vi "전체적인 좌표변환 구조.vi"() -> ()   [LabVIEW 2016]
panel:
  out "Lane":dbl[][](array[numeric])
  out "Obstacle":dbl[][](array[numeric])
  in  "IMU Data":string
  in  "Platform Data":string
  in  "NMEA Data":string
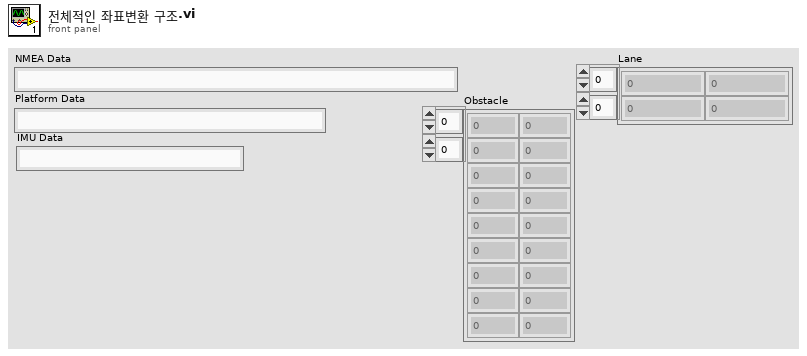
[diagram p1: front panel]
types:
  T1 = cluster{"GPS_Time":string, "GPS_Date":string, "GPS_N/S":string, "GPS_E/W":string, "GPS Raw_Lat":dbl, "GPS Raw_Lon":dbl, "GPS Raw_Speed [m/s]":dbl, "GPS Raw_Speed [km/h]":dbl, "GPS Raw_Bearing angle":dbl, "Checksum":bool, "Validity":bool}
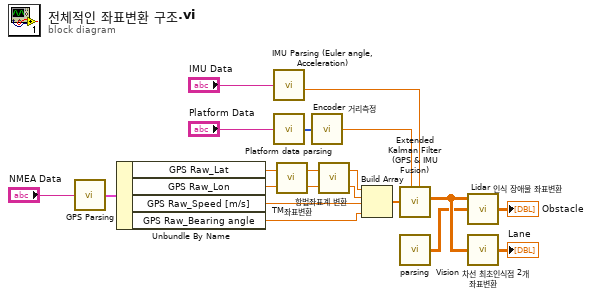
[diagram p0: block diagram]
diagram:
  n1 = call "GPS Parsing.vi"("NMEA Data"="NMEA Data") -> ("출력 클러스터"=w20:T1)
  n2 = Unbundle By Name(w20) -> ("GPS Raw_Lat"=w19:dbl, "GPS Raw_Lon"=w18:dbl, "GPS Raw_Speed [m/s]"=w3:dbl, "GPS Raw_Bearing angle"=w2:dbl)
  n3 = call "IMU Parsing (Euler angle, Acceleration).vi"("IMU Data"="IMU Data") -> ("IMU_Yaw"=w10:dbl)  [unwired: 4 in, 3 out]
  n4 = call "Platform data parsing.vi"("Platform Data"="Platform Data") -> ("Platform Data"=w14:u32[])
  n5 = call "TM좌표변환.vi"("lon"=w18, "lat"=w19) -> ("Y_TM"=w16:dbl, "X_TM"=w17:dbl)
  n6 = call "Encoder 거리측정.vi"("배열"=w14) -> ("Encoder_Speed"=w15:dbl)
  n7 = call "항법좌표계 변환.vi"("Y_TM"=w16, "X_TM"=w17) -> ("Y_Nav"=w4:dbl, "X_Nav"=w5:dbl)
  n8 = Build Array(w5, w4, w3, w2) -> (w1:dbl[])
  n9 = call "Extended Kalman Filter (GPS & IMU Fusion).vi"("theta_IMU"=w10, "v_Encoder"=w15, "X_GPS Raw"=w1) -> ("X"=w8:dbl[][])  [unwired: 8 in]
  n10 = call "parsing.vi"() -> ("배열"=w6:dbl[][])  [unwired: 1 in]
  n11 = call "Lidar 인식 장애물 좌표변환.vi"("Lidar"=w6, "GPS"=w8) -> ("Obstacle"=→"Obstacle":dbl[][])  [unwired: 1 in]
  n12 = call "Vision 차선 최초인식점 2개 좌표변환.vi"("GPS"=w8) -> ("Lane"=→"Lane":dbl[][])  [unwired: 2 in]
